vi "pmu_Build Data Width.vi"(8 "error in (no error)":errorcluster, 11 "system info in":refnum<class "PMU System Info.lvclass">) -> (0 "error out":errorcluster, 2 "init meas data":u8[](array[numeric]), 3 "system info out":refnum<class "PMU System Info.lvclass">)   [LabVIEW 2011, in "NI_EP_PMU.lvlib"]
uses:
  <vilib>/addons/Electrical Power/PMU/NI_EP_PMU.lvlib
  <vilib>/addons/Electrical Power/PMU/Common/Classes/PMU System Info/PMU System Info.lvclass
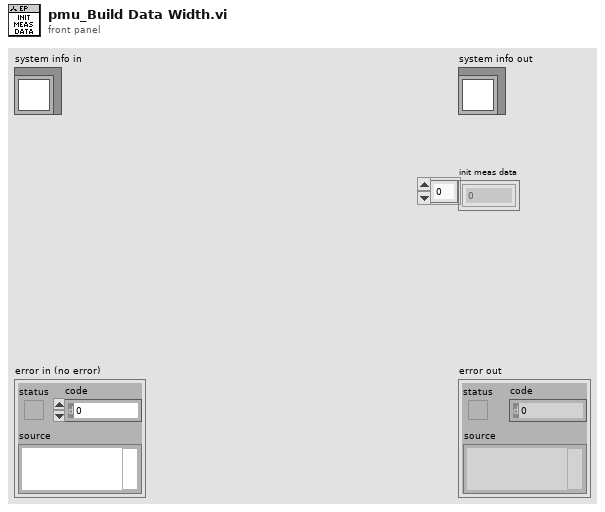
[diagram p1: front panel]
types:
  T1 = typedef "NI_EP_PMU.lvlib/pmu_CFG Class.ctl" = cluster{"station name":string, "PMU ID":u16, "time base":u32, "nominal frequency":enum16{"50 Hz", "60 Hz"}, "reporting rate":i16, "phasor number":u16, "analog number":u16, "digital number":u16, "channel names":string[], "phasor units":u32[], "analog units":u32[], "digital units":u32[], "data format":u16, "number of PMUs":u16}
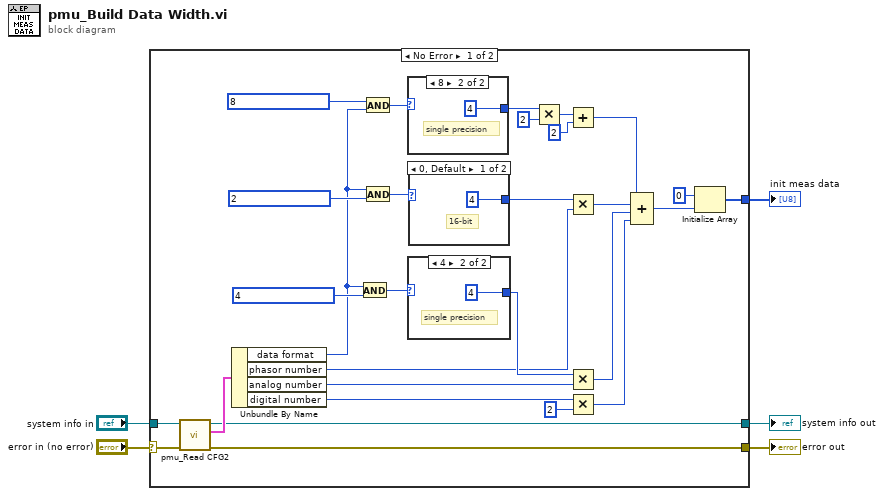
[diagram p0: block diagram]
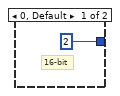
[diagram p2: hidden frame]
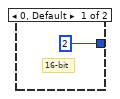
[diagram p3: hidden frame]
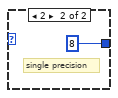
[diagram p4: hidden frame]
diagram:
  n1 = case shown="No Error" "error in (no error)" {
    selector: "error in (no error)" -> [w9 w41]
    tunnel: "system info in" -> [w24 w42]
    tunnel: [w11 w41] -> w4
    tunnel: [w10 w42] -> w3
    tunnel: [w6 _] -> w1
    frame No Error {
      n2 = call <vilib>:"pmu_Read CFG2.vi"("error in (no error)"=w9, "system info in"=w24) -> ("error out"=w11:errorcluster, "CFG-2"=w23:T1, "system info out"=w10:refnum<class "PMU System Info.lvclass">)  [unwired: 7 in]
      n3 = Unbundle By Name(w23) -> ("data format"=w22:u16, "phasor number"=w18:u16, "analog number"=w21:u16, "digital number"=w17:u16)
      n4 = And(x=w22, y=u16 4 ("x")) -> (x .and. y?=w31:u16)
      n5 = And(x=u16 8, y=w22) -> (x .and. y?=w29:u16)
      n6 = And(x=w22, y=u16 2 ("x")) -> (x .and. y?=w33:u16)
      n7 = case shown="8" w29 {
        tunnel: [u16 2 u16 4] -> w28
        frame 0, Default {
          # "16-bit"
        }
        frame 8 {
          # "single precision"
        }
      }
      n8 = case shown="4" w31 {
        tunnel: [u16 2 u16 4] -> w20
        frame 0, Default {
          # "16-bit"
        }
        frame 4 {
          # "single precision"
        }
      }
      n9 = case shown="0, Default" w33 {
        tunnel: [u16 4 u16 8] -> w19
        frame 0, Default {
          # "16-bit"
        }
        frame 2 {
          # "single precision"
        }
      }
      n10 = Multiply(x=w28, y=u16 2) -> (x*y=w26:u16)
      n11 = Add(x=w26, y=u16 2) -> (x+y=w15:u16)
      n12 = Multiply(x=w19, y=w18) -> (x*y=w14:u16)
      n13 = Multiply(x=w20, y=w21) -> (x*y=w12:u16)
      n14 = Multiply(x=w17, y=u16 2) -> (x*y=w13:u16)
      n15 = Compound Arithmetic op=ADD(w15, w14, w12, w13) -> (w8:u16)
      n16 = Initialize Array(u8 0 ("element"), w8) -> (w6:u8[])
    }
    frame Error {
    }
  }
  "error out" <- w4
  "system info out" <- w3
  "init meas data" <- w1
